vi "1C Camera Interpreter.vi"() -> (0 "error out":errorcluster, 1 "Overhead Image":T1(plugin-control), 2 "Heading":T2 format="%05.1f", 3 "Boat Location":T3 {"North" format="%#_10f"; "East" format="%#_8f"}, 4 "Time Elapsed (s)\nSince Last Image":dbl)   [LabVIEW 2011]
doc: "Using data from a cameram, attempts to track two fiducial patterns on the boat, one on the bow and one on the stern. Uses these positions to estimate boat position in the pool.\n\noptimizations for speed: \n-uses an oval-shaped mask to search for the tracking patterns only inside the pool\n-runs the two pattern searches separately so that they can be parallelized\n-upgraded to larger patterns\n\nBy: Cory Dolphin, Jason Curtis, Gray Thomas"
uses:
  <vilib>/userdefined/High Color/IMAQdx.ctl
  2-Think/2 Typedefs/UTM Location.ctl
  2-Think/2 Typedefs/heading.ctl
  2-Think/2 Typedefs/indicator LED.ctl
  2-Think/2 Globals/2 Global.vi
  <vilib>/vision/driver/NI_Vision_Acquisition_Software.lvlib
panel:
  in  "Image Descriptor Path":path=path "../../1,3 C-Small RC Platform/LPB Pool Image Descriptor.txt"
  out "Masked image":T1(plugin-control)
  in  "Minimum Stern Match Score":sgl=650.0
  in  "Minimum Bow Match Score":sgl=850.0
  in  "Reset Camera":bool
  in  "Camera Selector":T4="cam7"
  # "(ignore UTM Zone \nand Hemisphere for \nRC boat)"
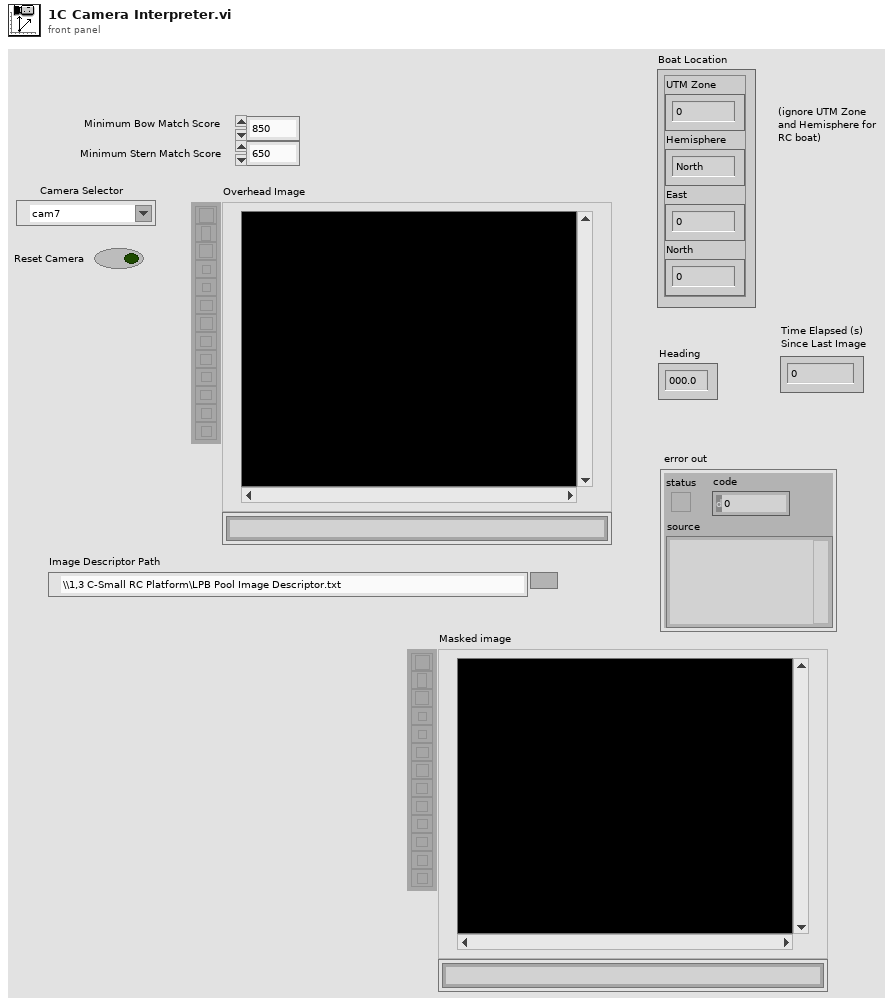
[diagram p1: front panel]
types:
  T1 = typedef "IMAQ Image.ctl" = refnum<image>
  T2 = typedef "heading.ctl" = dbl
  T3 = typedef "UTM Location.ctl" = cluster{"UTM Zone":dbl, "Hemisphere":enum16{"North", "South"}, "East":dbl, "North":dbl}
  T4 = typedef "IMAQdx.ctl" = refnum<k21>
  T5 = typedef "Image Type" = u32
  T6 = typedef "indicator LED.ctl" = bool
  T7 = typedef "0-Image Descriptor.ctl" = cluster{"Upper-Left Corner Coordinates":T3, "Meters/Pixel":dbl}
  T8 = typedef "generalized sensor status.ctl" = cluster{"Sensor Connected":T6, "Sensor Initialized":T6, "Sensor OK":T6, "Latest Error String":string, "GPS Lock":T6}
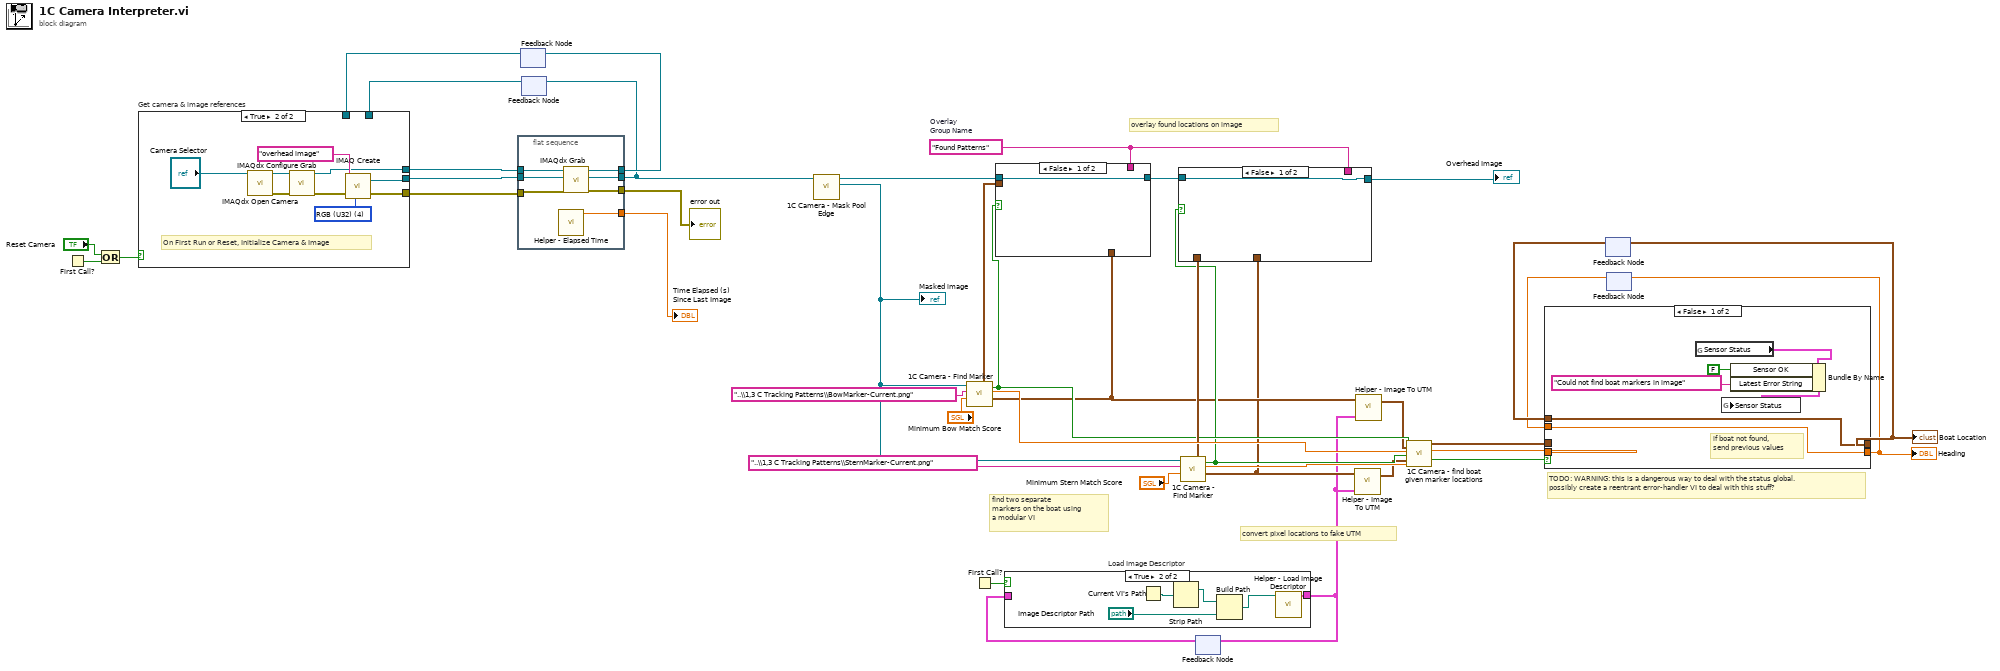
[diagram p0: block diagram]
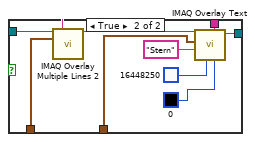
[diagram p3: hidden frame]
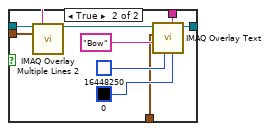
[diagram p4: hidden frame]
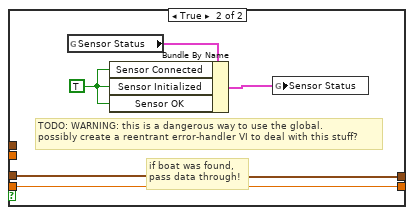
[diagram p5: hidden frame]
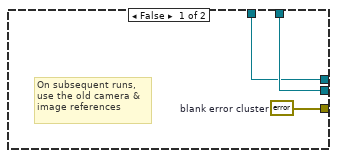
[diagram p6: hidden frame]
diagram:
  w14 = "Found Patterns"  # Overlay Group Name
  # "find two separate\nmarkers on the boat using \na modular VI"
  # "TODO: WARNING: this is a dangerous way to deal with the status global. \npossibly create a reentrant error-handler VI to deal with this stuff?"
  # "convert pixel locations to fake UTM"
  # "overlay found locations on image"
  n1 = First Call?() -> (First Call?: T/F=w40:bool)
  n2 = Or(x="Reset Camera", y=w40) -> (x .or. y?=w33:bool)
  n3 = flat-sequence {
    tunnel: [w48] -> w41
    tunnel: w39 -> [w47]
    tunnel: w38 -> [w46]
    tunnel: w37 -> [w45]
    tunnel: [w44] -> w36
    tunnel: [w43] -> w21
    tunnel: [w42] -> w13
    frame #0 {
      n4 = call "Helper - Elapsed Time.vi"() -> ("Time Elapsed (s)\nSince Last Iteration"=w42:dbl)  [unwired: 10 in, 1 out]
      n5 = call <vilib>:"IMAQdx Grab.vi"("error in"=w46, "Image In"=w45, "Session In"=w47) -> ("error out"=w48:errorcluster, "Image Out"=w43:T1, "Session Out"=w44:T4)  [unwired: 5 in, 1 out]
    }
  }
  n6 = feedback #1() -> (w34:T4)  [unwired: 1 in]
  n7 = feedback-in #1(w36) -> ()
  n8 = feedback-in #2(w21) -> ()
  n9 = feedback #2() -> (w35:T1)  [unwired: 1 in]
  n10 = case "Get camera & image references" shown="True" w33 {
    tunnel: [w50 w54] -> w39
    tunnel: [w49 w53] -> w38
    tunnel: [w51 w52] -> w37
    tunnel: w35 -> [w51 _]
    tunnel: w34 -> [w50 _]
    frame False {
      w49 = errorcluster {"status"=FALSE, "code"=0, "source"=""}  # blank error cluster
      # "On subsequent runs,\nuse the old camera &\nimage references"
    }
    frame True {
      w56 = T5 4 items=["Grayscale (U8)", "Grayscale (I16)", "Grayscale (SGL)", "Complex (CSG)", "RGB (U32)", "HSL (U32)", "RGB (U64)", "Grayscale (U16)"] ("Image Type")
      # "On First Run or Reset, Initialize Camera & Image"
      n11 = call <vilib>:"IMAQdx Open Camera.vi"("Session In"="Camera Selector") -> ("error out"=w57:errorcluster, "Session Out"=w60:T4)  [unwired: 9 in]
      n12 = call <vilib>:"IMAQdx Configure Grab.vi"("error in"=w57, "Session In"=w60) -> ("error out"=w58:errorcluster, "Session Out"=w54:T4)  [unwired: 8 in]
      n13 = call "IMAQ Create"("Image Name"="overhead image", "Image Type"=w56, "error in (no error)"=w58) -> ("New Image"=w52:T1, "error out"=w53:errorcluster)  [unwired: 2 in]
    }
  }
  n14 = call "1C Camera - Mask Pool Edge.vi"("Source Image In"=w21) -> ("Masked Image Out"=w8:T1, "Src Image Out"=w20:T1)  [unwired: 9 in]
  "Masked image" <- w8
  n15 = call "1C Camera - Find Marker.vi"("Minimum Match Score (650)"="Minimum Bow Match Score", "marker template relative path"="..\\1,3 C Tracking Patterns\\BowMarker-Current.png", "Image In"=w8) -> ("Best Match Position"=w5:cluster{"x":sgl, "y":sgl}, "Best Match Heading"=w31:T2, "Best Match\nBounding Box"=w18:cluster{"x":sgl, "y":sgl}[], "Marker found?"=w12:T6)  [unwired: 3 in, 2 out]
  n16 = First Call?() -> (First Call?: T/F=w3:bool)
  n17 = case shown="False" w12 {
    tunnel: w20 -> [w61 w67]
    tunnel: w5 -> [_ w66]
    tunnel: w18 -> [_ w64]
    tunnel: [w61 w63] -> w17
    tunnel: w14 -> [_ w62]
    frame False {
    }
    frame True {
      n18 = call "IMAQ Overlay Multiple Lines 2"("Image"=w67, "Group"=w62, "Line End Points"=w64) -> ("Image Out"=w65:T1)  [unwired: 11 in, 1 out]
      n19 = call "IMAQ Overlay Text"("BG Color (Transparent)"=u32 0, "Group"=w62, "Text Color (black)"=u32 16448250, "String"="Bow", "Origin"=w66, "Image"=w65) -> ("Image Out"=w63:T1)  [unwired: 4 in, 1 out]
    }
  }
  n20 = call "1C Camera - Find Marker.vi"("Minimum Match Score (650)"="Minimum Stern Match Score", "marker template relative path"="..\\1,3 C Tracking Patterns\\SternMarker-Current.png", "Image In"=w8) -> ("Best Match Position"=w4:cluster{"x":sgl, "y":sgl}, "Best Match Heading"=w19:T2, "Best Match\nBounding Box"=w16:cluster{"x":sgl, "y":sgl}[], "Marker found?"=w11:T6)  [unwired: 3 in, 2 out]
  n21 = case shown="False" w11 {
    tunnel: w4 -> [_ w77]
    tunnel: w17 -> [w71 w76]
    tunnel: w16 -> [_ w74]
    tunnel: [w71 w73] -> w15
    tunnel: w14 -> [_ w72]
    frame False {
    }
    frame True {
      n22 = call "IMAQ Overlay Multiple Lines 2"("Image"=w76, "Group"=w72, "Line End Points"=w74) -> ("Image Out"=w75:T1)  [unwired: 11 in, 1 out]
      n23 = call "IMAQ Overlay Text"("BG Color (Transparent)"=u32 0, "Group"=w72, "Text Color (black)"=u32 16448250, "String"="Stern", "Origin"=w77, "Image"=w75) -> ("Image Out"=w73:T1)  [unwired: 4 in, 1 out]
    }
  }
  "Overhead Image" <- w15
  n24 = feedback #3() -> (w2:T7)  [unwired: 1 in]
  n25 = case "Load Image Descriptor" shown="True" w3 {
    tunnel: [w81 w86] -> w1
    tunnel: w2 -> [w81 _]
    frame False {
    }
    frame True {
      n26 = Current VI's Path() -> (path=w84:path)
      n27 = Strip Path(path=w84) -> (stripped path=w83:path)  [unwired: 1 out]
      n28 = Build Path(base path=w83, name or relative path="Image Descriptor Path") -> (appended path=w82:path)
      n29 = call "Helper - Load Image Descriptor.vi"("Image Descriptor File Path"=w82) -> ("Image Descriptor Typedef out"=w86:T7)  [unwired: 10 in]
    }
  }
  n30 = feedback-in #3(w1) -> ()
  n31 = call "Helper - Image To UTM.vi"("Image Descriptor"=w1, "Pixel Coordinates"=w4) -> ("UTM Location"=w6:T3)  [unwired: 1 in, 1 out]
  n32 = call "Helper - Image To UTM.vi"("Image Descriptor"=w1, "Pixel Coordinates"=w5) -> ("UTM Location"=w7:T3)  [unwired: 1 in, 1 out]
  n33 = call "1C Camera - find boat given marker locations.vi"("Bow Marker Found"=w12, "Bow Marker Location"=w7, "Bow Marker Heading"=w31, "Stern Marker Found"=w11, "Stern Marker Location"=w6, "Stern Marker Heading"=w19) -> ("Boat Location"=w29:T3, "Heading"=w28:T2, "Boat Found"=w30:T6)  [unwired: 11 in]
  n34 = feedback #4() -> (w26:T3)  [unwired: 1 in]
  n35 = feedback #5() -> (w24:T2)  [unwired: 1 in]
  n36 = case shown="False" w30 {
    tunnel: [w92 w97] -> w27
    tunnel: w29 -> [_ w97]
    tunnel: [w91 w96] -> w25
    tunnel: w28 -> [_ w96]
    tunnel: w26 -> [w92 _]
    tunnel: w24 -> [w91 _]
    frame False {
      # "if boat not found,\nsend previous values"
      n37 = global read "2 Global.vi" "Sensor Status"() -> (w90:T8)
      n38 = Bundle By Name(cluster=w90, "Sensor OK"=T6 FALSE, "Latest Error String"="Could not find boat markers in image" ("Error String")) -> (w87:T8)
      n39 = global write "2 Global.vi" "Sensor Status"(w87) -> ()
    }
    frame True {
      w93 = T6 TRUE ("Sensor OK")
      # "TODO: WARNING: this is a dangerous way to use the global. \npossibly create a reentrant error-handler VI to deal with this stuff?"
      # "if boat was found, \npass data through!"
      n40 = global read "2 Global.vi" "Sensor Status"() -> (w95:T8)
      n41 = Bundle By Name(cluster=w95, "Sensor Connected"=w93, "Sensor Initialized"=w93, "Sensor OK"=w93) -> (w94:T8)
      n42 = global write "2 Global.vi" "Sensor Status"(w94) -> ()
    }
  }
  "Boat Location" <- w27
  "Heading" <- w25
  n43 = feedback-in #4(w27) -> ()
  n44 = feedback-in #5(w25) -> ()
  "error out" <- w41
  "Time Elapsed (s)\nSince Last Image" <- w13
